vi "lvclass to string files.vi"(4 "Export Diagram":bool, 6 "Create Captions":bool=TRUE, 8 "error in (no error)":errorcluster, 10 "Class String Files Root":path=path "E:/VI2String/Test Project/Test Project.lvproj", 11 "lvclass Path":path) -> (0 "error out":errorcluster)   [LabVIEW 2022 SP3]
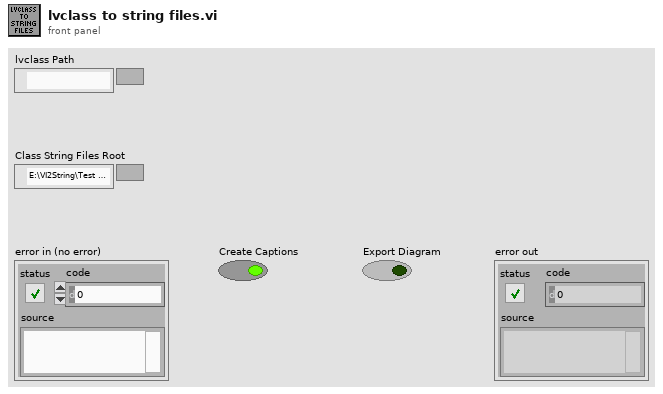
[diagram p1: front panel]
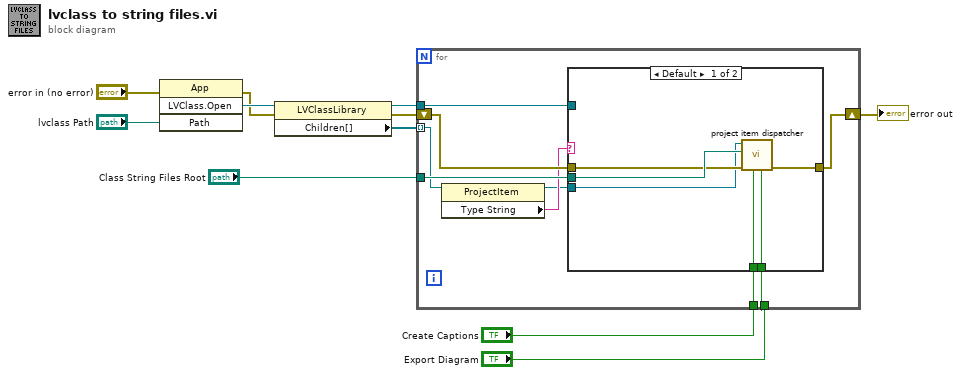
[diagram p0: block diagram]
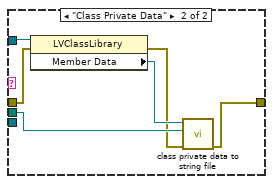
[diagram p2: hidden frame]
diagram:
  n1 = invoke class="App" method="LVClass.Open"(error in="error in (no error)", "Path"="lvclass Path") -> (error out=w5:errorcluster, "LVClass.Open"=w11:refnum<vi>)  [unwired: 2 in, 2 out]
  n2 = property class="LVClassLibrary"(reference=w11, error in=w5) -> (reference out=w2:refnum<vi>, error out=w4:errorcluster, "Children[]"=w10:refnum<vi>[])
  n3 = for {
    tunnel: w10 -> [w15] mode=indexing
    tunnel: "Create Captions" -> [w20]
    tunnel: "Export Diagram" -> [w19]
    tunnel: "Class String Files Root" -> [w18]
    shift-right: [w16] -> w3
    shift-left: w4 -> [w17]
    tunnel: w2 -> [w13]
    n4 = property class="ProjectItem"(reference=w15) -> (reference out=w12:refnum<vi>, "Type String"=w14:string)  [unwired: 1 in, 1 out]
    n5 = case shown="Default" w14 {
      tunnel: w20 -> [w26 _]
      tunnel: w19 -> [w25 _]
      tunnel: w18 -> [w24 w32]
      tunnel: w17 -> [w23 w28]
      tunnel: [w22 w31] -> w16
      tunnel: w13 -> [_ w30]
      tunnel: w12 -> [w21 _]
      frame Default {
        n6 = call "project item dispatcher.vi"("Export Diagram"=w25, "Create Captions"=w26, "error in (no error)"=w23, "String Files Root"=w24, "ProjectItem in"=w21) -> ("error out"=w22:errorcluster)  [unwired: 6 in]
      }
      frame "Class Private Data" {
        n7 = property class="LVClassLibrary"(reference=w30, error in=w28) -> (error out=w27:errorcluster, "Member Data"=w29:refnum<vi>)  [unwired: 1 out]
        n8 = call "class private data to string file.vi"("error in (no error)"=w27, "String Files Root"=w32, "Private Data Control"=w29) -> ("error out"=w31:errorcluster)  [unwired: 8 in]
      }
    }
  }
  "error out" <- w3
